vi "StarTrekIndicator.vi"(4 "in":bool[](array[boolean])) -> (1 "out":bool[](array[boolean]))   [LabVIEW 2016]
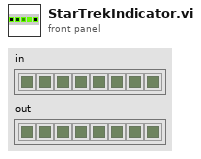
[diagram p1: front panel]
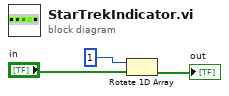
[diagram p0: block diagram]
diagram:
  n1 = Rotate 1D Array(1:"in", 2:1 ("n")) -> (0:→"out":bool[])
